vi "Update Monitor.QueueSize by ID.vi"(7 "PackageID":i32, 8 "error in":errorcluster, 11 "Queue Size":u32) -> (0 "error out":errorcluster)   [LabVIEW 2021, in "XNET-CAN-Signal-Logger.lvlib"]
uses:
  XNET-CAN-Signal-Logger.lvlib
  Global Variables.vi
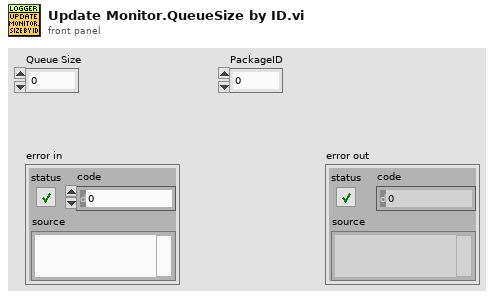
[diagram p1: front panel]
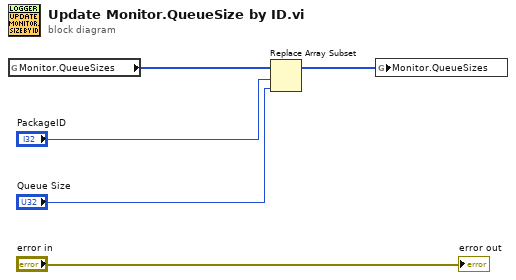
[diagram p0: block diagram]
diagram:
  n1 = global read "Global Variables.vi" "Monitor.QueueSizes"() -> (w5:u32[])
  n2 = Replace Array Subset(array=w5, new element="Queue Size", index="PackageID") -> (w3:u32[])
  n3 = global write "Global Variables.vi" "Monitor.QueueSizes"(w3) -> ()
  "error out" <- "error in"
